vi "FindEngResultsFile.vi"(0 "Input Path":path, 1 "EEPROM Template File":string, 2 "Eng-Results":u32, 3 "Create Eng Results File?":bool, 4 "Re Create Eng Results File?":bool) -> (7 "Engr Result File":path)   [LabVIEW 2015]
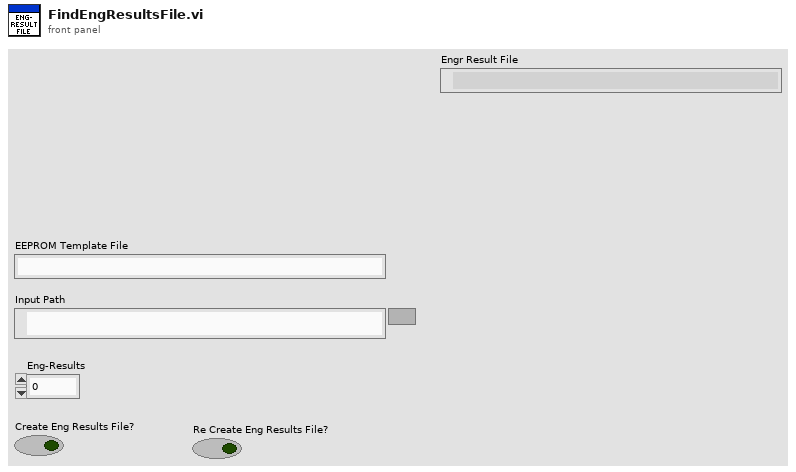
[diagram p1: front panel]
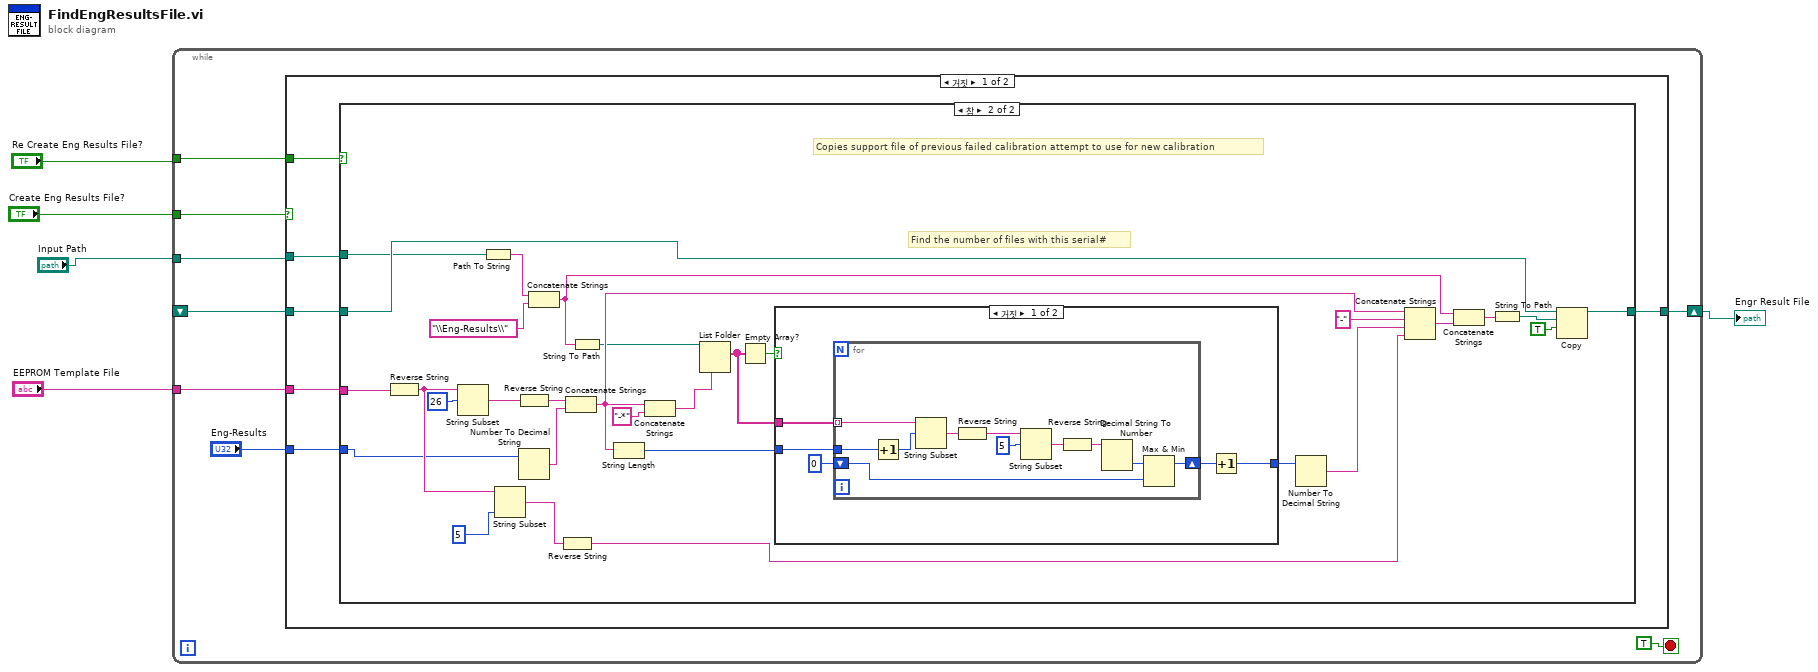
[diagram p0: block diagram]
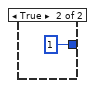
[diagram p3: hidden frame]
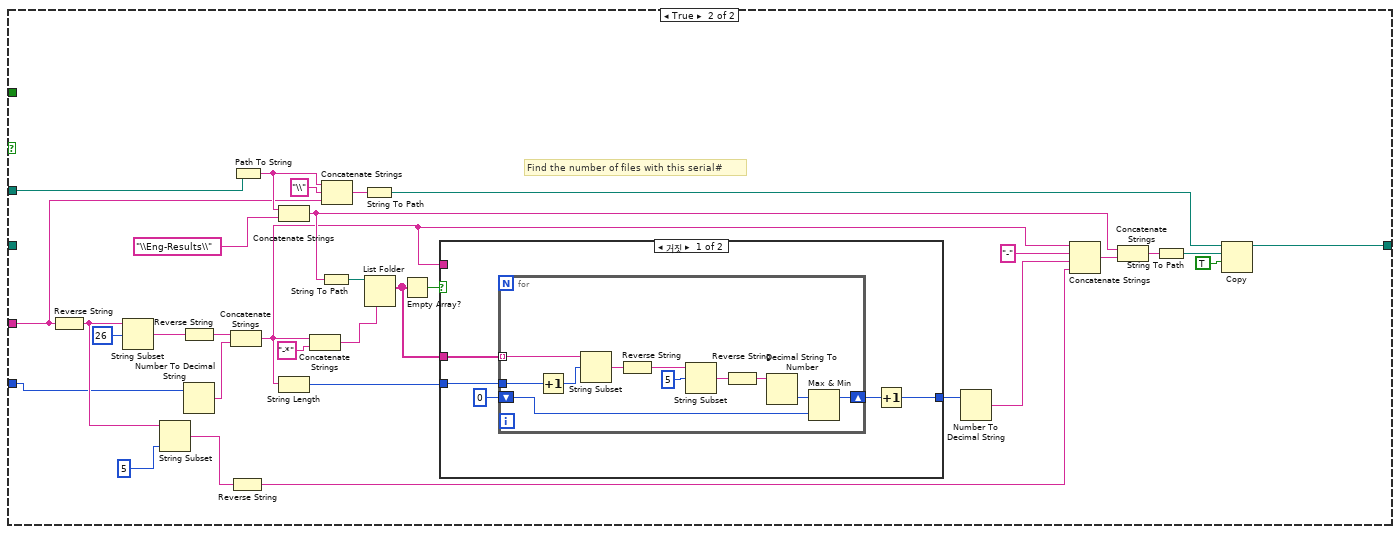
[diagram p4: hidden frame]
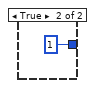
[diagram p5: hidden frame]
diagram:
  n1 = while {
    tunnel: "Create Eng Results File?" -> [w12]
    tunnel: "EEPROM Template File" -> [w11]
    tunnel: "Input Path" -> [w10]
    shift-right: [w9] -> w2
    shift-left: _ -> [w8]
    tunnel: "Re Create Eng Results File?" -> [w7]
    stop <- TRUE stop-if-true
    n2 = case shown="거짓" w12 {
      tunnel: w11 -> [w16 w71]
      tunnel: w10 -> [w17 w98]
      tunnel: [w18 w80] -> w9
      tunnel: w8 -> [w19 _]
      tunnel: w7 -> [w15 _]
      tunnel: "Eng-Results" -> [w14 w68]
      frame False {
        n3 = case shown="참" w15 {
          tunnel: w19 -> [w20 w28]
          tunnel: [w20 w27] -> w18
          tunnel: w17 -> [_ w26]
          tunnel: w16 -> [_ w23]
          tunnel: w14 -> [_ w21]
          frame False {
          }
          frame True {
            # "Copies support file of previous failed calibration attempt to use for new calibration"
            # "Find the number of files with this serial#"
            n4 = Reverse String(1:w23) -> (0:w46:string)
            n5 = String Subset(string=w46, offset (0)=26) -> (substring=w31:string)  [unwired: 1 in]
            n6 = Path To String(path=w26) -> (string=w48:string)
            n7 = String Subset(string=w46, length (rest)=5 ("offset (0)")) -> (substring=w45:string)  [unwired: 1 in]
            n8 = Reverse String(1:w31) -> (0:w33:string)
            n9 = Number To Decimal String(number=w21) -> (decimal integer string=w29:string)  [unwired: 1 in]
            n10 = Concatenate Strings(w48, "\\Eng-Results\\") -> (w22:string)
            n11 = Reverse String(1:w45) -> (0:w47:string)
            n12 = Concatenate Strings(w33, w29) -> (w42:string)
            n13 = String To Path(string=w22) -> (path=w24:path)
            n14 = String Length(string=w42) -> (length=w43:i32)
            n15 = Concatenate Strings(w42, "-*" ("string")) -> (w35:string)
            n16 = List Folder(path=w24, pattern=w35) -> (filenames=w40:string[])  [unwired: 2 in, 3 out]
            n17 = Empty Array?(array=w40) -> (empty?=w41:bool)
            n18 = case shown="거짓" w41 {
              tunnel: [w55 u32 1 ("output 1")] -> w30
              tunnel: w40 -> [w54 _]
              tunnel: w43 -> [w53 _]
              frame False {
                n19 = for {
                  tunnel: w54 -> [w60] mode=indexing
                  tunnel: w53 -> [w66]
                  shift-right: [w57] -> w52
                  shift-left: 0 -> [w56]
                  n20 = Increment(x=w66) -> (x+1=w65:i32)
                  n21 = String Subset(string=w60, offset (0)=w65) -> (substring=w64:string)  [unwired: 1 in]
                  n22 = Reverse String(1:w64) -> (0:w63:string)
                  n23 = String Subset(string=w63, offset (0)=5) -> (substring=w61:string)  [unwired: 1 in]
                  n24 = Reverse String(1:w61) -> (0:w59:string)
                  n25 = Decimal String To Number(string=w59) -> (number=w58:i32)  [unwired: 2 in, 1 out]
                  n26 = Max & Min(x=w58, y=w56) -> (max(x,y)=w57:i32)  [unwired: 1 out]
                }
                n27 = Increment(x=w52) -> (x+1=w55:i32)
              }
              frame True {
              }
            }
            n28 = Number To Decimal String(number=w30) -> (decimal integer string=w39:string)  [unwired: 1 in]
            n29 = Concatenate Strings(w42, "-" ("string"), w39, w47) -> (w49:string)
            n30 = Concatenate Strings(w22, w49) -> (w50:string)
            n31 = String To Path(string=w50) -> (path=w37:path)
            n32 = Copy(9:TRUE ("overwrite (F)"), 10:w37, 11:w28) -> (3:w27:path)  [unwired: 2 in, 2 out]
          }
        }
      }
      frame True {
        # "Find the number of files with this serial#"
        n33 = Reverse String(1:w71) -> (0:w70:string)
        n34 = String Subset(string=w70, offset (0)=26) -> (substring=w94:string)  [unwired: 1 in]
        n35 = String Subset(string=w70, length (rest)=5 ("offset (0)")) -> (substring=w72:string)  [unwired: 1 in]
        n36 = Reverse String(1:w94) -> (0:w92:string)
        n37 = Number To Decimal String(number=w68) -> (decimal integer string=w99:string)  [unwired: 1 in]
        n38 = Concatenate Strings(w92, w99) -> (w75:string)
        n39 = Reverse String(1:w72) -> (0:w69:string)
        n40 = Path To String(path=w98) -> (string=w82:string)
        n41 = Concatenate Strings(w82, "\\Eng-Results\\") -> (w86:string)
        n42 = String Length(string=w75) -> (length=w74:i32)
        n43 = Concatenate Strings(w75, "-*" ("string")) -> (w90:string)
        n44 = String To Path(string=w86) -> (path=w96:path)
        n45 = Concatenate Strings(w82, "\\" ("string"), w71) -> (w88:string)
        n46 = String To Path(string=w88) -> (path=w87:path)
        n47 = List Folder(path=w96, pattern=w90) -> (filenames=w77:string[])  [unwired: 2 in, 3 out]
        n48 = Empty Array?(array=w77) -> (empty?=w76:bool)
        n49 = case shown="거짓" w76 {
          tunnel: [w104 u32 1 ("output 1")] -> w95
          tunnel: w75 -> [_ _]
          tunnel: w77 -> [w103 _]
          tunnel: w74 -> [w102 _]
          frame False {
            n50 = for {
              tunnel: w103 -> [w109] mode=indexing
              tunnel: w102 -> [w115]
              shift-right: [w106] -> w101
              shift-left: 0 -> [w105]
              n51 = Increment(x=w115) -> (x+1=w114:i32)
              n52 = String Subset(string=w109, offset (0)=w114) -> (substring=w113:string)  [unwired: 1 in]
              n53 = Reverse String(1:w113) -> (0:w112:string)
              n54 = String Subset(string=w112, offset (0)=5) -> (substring=w110:string)  [unwired: 1 in]
              n55 = Reverse String(1:w110) -> (0:w108:string)
              n56 = Decimal String To Number(string=w108) -> (number=w107:i32)  [unwired: 2 in, 1 out]
              n57 = Max & Min(x=w107, y=w105) -> (max(x,y)=w106:i32)  [unwired: 1 out]
            }
            n58 = Increment(x=w101) -> (x+1=w104:i32)
          }
          frame True {
          }
        }
        n59 = Number To Decimal String(number=w95) -> (decimal integer string=w78:string)  [unwired: 1 in]
        n60 = Concatenate Strings(w75, "-" ("string"), w78, w69) -> (w85:string)
        n61 = Concatenate Strings(w86, w85) -> (w84:string)
        n62 = String To Path(string=w84) -> (path=w83:path)
        n63 = Copy(9:TRUE ("overwrite (F)"), 10:w83, 11:w87) -> (3:w80:path)  [unwired: 2 in, 2 out]
      }
    }
  }
  "Engr Result File" <- w2
